vi "参数.vi"() -> ()   [LabVIEW 2018]
uses:
  <vilib>/vision/Image Controls.llb/IMAQ Image.ctl
panel:
  in  "测量停止":bool
  in  "系统运行状态":enum16{"通信测试", "初始化", "测量", "写入"}(ring)
  in  "当前测量状态":T1(ring)
  in  "激光器状态":T2
  out "本次任务":T3
  in  "全局关机":bool
  in  "ErrorLog":string
  out "运行参数":T5={"示波器"={"Channel (0:Channel 1)"=enum."Channel 1", "电压范围"=0.0, "触发电压"=0.0, "时间范围"=0.0, " 示波器VISA"=""}, "光谱仪"={"Channel (0:Channel 1)"=enum."Channel 1", "电压范围"=0, "触发电压"=0, "时间范围"=0}, " 近场相机"={"曝光时间"=0, "模拟增益"=0, "控制套接字"=0, "IP 地址"="", " 采集套接字"=0, "  版本号"=0, "ImageData"=refnum, "  增益最大"=0, "  增益最小"=0, " 曝光最大"=0, " 曝光最小"=0, " 帧速"=0, " 同步切换"=0, "  曝光缩放"=0}, " 偏振仪"={"电压范围"=0, "触发电压"=0, "时间范围"=0, "波长范围"=enum."可见光 400-700nm"}, " 功率计"={"通道"=enum."Channel 1", "工作波长"=0, "单位"=0, "时间范围"=0, "IP地址"="192.168.129.77", "端口"=4001}, "能量计"={"通道"=enum."Channel 1", "工作波长"=0, "单位"=0, "时间范围"=0, "IP地址"="192.168.129.77", "端口"=4001, "能量计量程"=enum."200uJ"}, "电机"={"Channel (0:Channel 1)"=enum."Channel 1", "电压范围"=0, "触发电压"=0, "时间范围"=0}, " 远场相机"={"曝光时间"=0, "模拟增益"=0, "控制套接字"=0, "IP 地址"="", " 采集套接字"=0, "  版本号"=0, "ImageData"=refnum, "  增益最大"=0, "  增益最小"=0, " 曝光最大"=0, " 曝光最小"=0, " 帧速"=0, " 同步切换"=0, "  曝光缩放"=0}}
  # "错误代码\n0 示波器初始化错误\n1 近场相机初始化错误\n2 能量功率表头初始化错误\n\n\n12 能量 测量错误\n13 功率 测量错误"
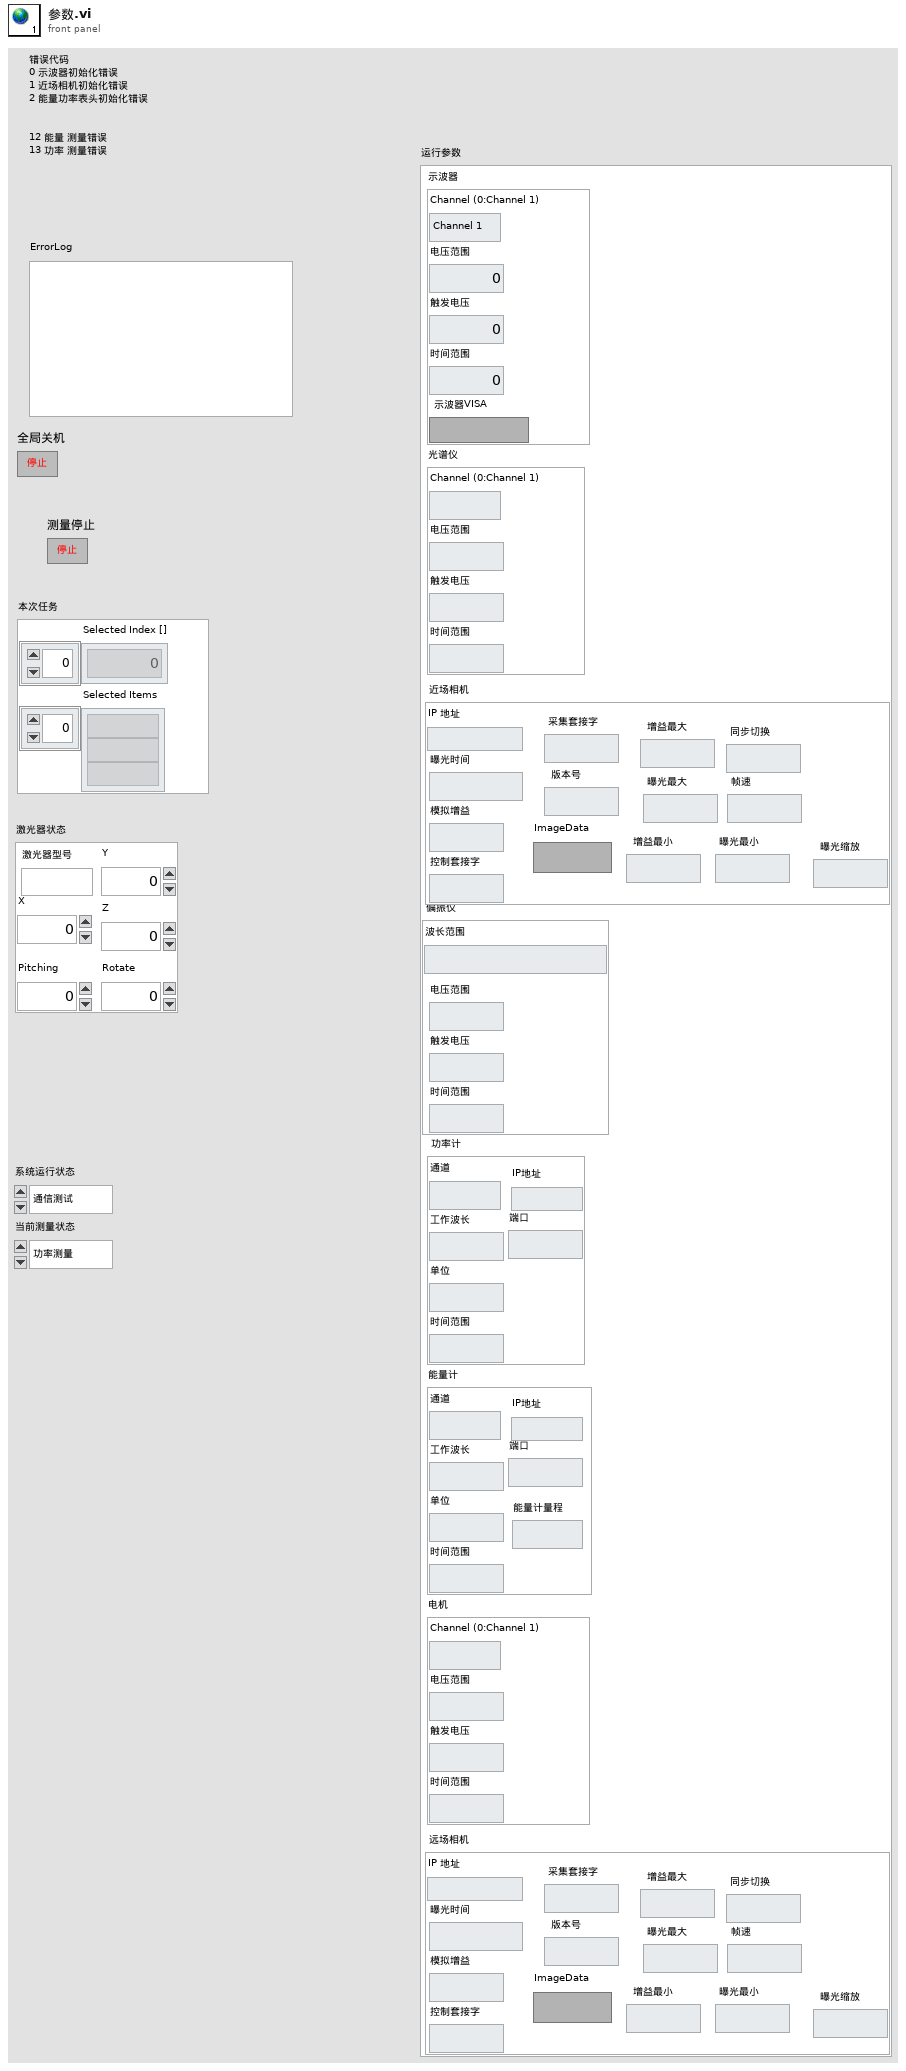
[diagram p1: front panel]
types:
  T1 = enum16{"功率测量", "能量测量", "光谱测量", "时间波形", "偏振测量", "近远场"}
  T2 = cluster{"激光器型号":string, "X":dbl, "Y":dbl, "Z":dbl, "Rotate":dbl, "Pitching":dbl}
  T3 = cluster{"Selected Index []":i32[], "Selected Items":string[]}
  T4 = typedef "IMAQ Image.ctl" = refnum<image>
  T5 = cluster{"示波器":cluster{"Channel (0:Channel 1)":enum16{"Channel 1", "Channel 2", "Channel 3", "Channel 4"}, "电压范围":dbl, "触发电压":dbl, "时间范围":dbl, " 示波器VISA":refnum<visa-resource-name>}, "光谱仪":cluster{"Channel (0:Channel 1)":enum16{"Channel 1", "Channel 2", "Channel 3", "Channel 4"}, "电压范围":u64, "触发电压":u64, "时间范围":u64}, " 近场相机":cluster{"曝光时间":i32, "模拟增益":i32, "控制套接字":i32, "IP 地址":string, " 采集套接字":i32, "  版本号":i32, "ImageData":T4, "  增益最大":i32, "  增益最小":i32, " 曝光最大":i32, " 曝光最小":i32, " 帧速":i32, " 同步切换":i32, "  曝光缩放":i32}, " 偏振仪":cluster{"电压范围":u64, "触发电压":u64, "时间范围":u64, "波长范围":enum16{"可见光 400-700nm", "近红外 700-1100nm"}}, " 功率计":cluster{"通道":enum16{"Channel 1", "Channel 2"}, "工作波长":u32, "单位":u64, "时间范围":u64, "IP地址":string, "端口":u32}, "能量计":cluster{"通道":enum16{"Channel 1", "Channel 2"}, "工作波长":u32, "单位":u64, "时间范围":u64, "IP地址":string, "端口":u32, "能量计量程":enum16{"200uJ", "20uJ", "2uJ", "200nJ"}}, "电机":cluster{"Channel (0:Channel 1)":enum16{"Channel 1", "Channel 2", "Channel 3", "Channel 4"}, "电压范围":u64, "触发电压":u64, "时间范围":u64}, " 远场相机":cluster{"曝光时间":i32, "模拟增益":i32, "控制套接字":i32, "IP 地址":string, " 采集套接字":i32, "  版本号":i32, "ImageData":T4, "  增益最大":i32, "  增益最小":i32, " 曝光最大":i32, " 曝光最小":i32, " 帧速":i32, " 同步切换":i32, "  曝光缩放":i32}}
diagram:
